vi "JSON to LVObject - Warning Input - Returns Same Warning.vi"() -> ()   [LabVIEW 2017, in "Generic Object Serializer Tests.lvlib"]
uses:
  Generic Object Serializer Tests.lvlib
  Generic Object Serializer/Generic Object Serializer.lvclass
  <vilib>/Utility/error.llb/Error Cluster From Error Code.vi
  <vilib>/addons/_JKI Toolkits/Caraya/classes/Assert/Assert Equal Value_Variant.vi
  <vilib>/ErrorRing/Error Ring.xnode
  <vilib>/addons/_JKI Toolkits/Caraya/classes/Test/Test.lvclass
  <vilib>/addons/_JKI Toolkits/Caraya/classes/Assert/Assert.lvclass
panel:
  out "error out":errorcluster
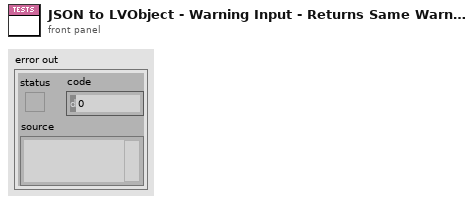
[diagram p1: front panel]
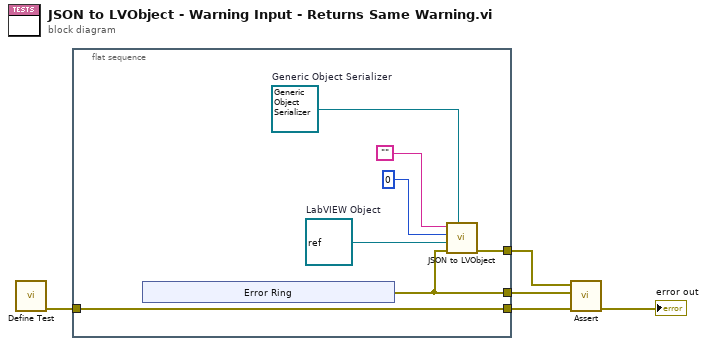
[diagram p0: block diagram]
diagram:
  n1 = call <vilib>:"Define Test.vi"() -> ("error out"=w4:errorcluster)  [unwired: 11 in]
  n2 = flat-sequence {
    tunnel: w4 -> [w10]
    tunnel: [w10] -> w3
    tunnel: [w9] -> w2
    tunnel: [w8] -> w1
    frame #0 {
      w11 = refnum<class> refnum  # LabVIEW Object
      w12 = refnum<class "Generic Object Serializer.lvclass"> refnum  # Generic Object Serializer
      n3 = xnode "Error Ring"() -> ("error out"=w8:errorcluster)
      n4 = call-dynamic "JSON to LVObject.vi"("LVClass Serializer"=w12, "error in (no error)"=w8, "Object Type"=w11, "Offset"=0, "JSON"="") -> ("error out"=w9:errorcluster)  [unwired: 5 in, 1 out]
    }
  }
  n5 = call-poly <vilib>:"Assert.vi"("error in (no error)"=w3, "Y"=w1, "X"=w2) -> ("error out"=→"error out":errorcluster)  [unwired: 8 in]
